vi "Get Tx IPs and Ports.vi"(0 "Target Names":string[](array[string])=["AE-HIL-1", "AE-HIL-2", "AE-HIL-3"], 1 "IP Addresses":string[](array[string])=["169.254.239.43", "169.254.184.119", "169.254.184.0"], 7 "Remote Target Name":string="AE-HIL-2", 13 "Local Target Index":i32) -> (4 "Local IP Address":string="169.254.239.43", 6 "Local Port Number":string="1000", 10 "Remote IP Address":string, 15 "Remote Port Number":string="1000")   [LabVIEW 2023]
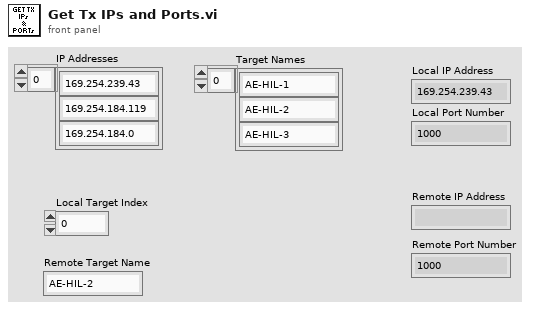
[diagram p1: front panel]
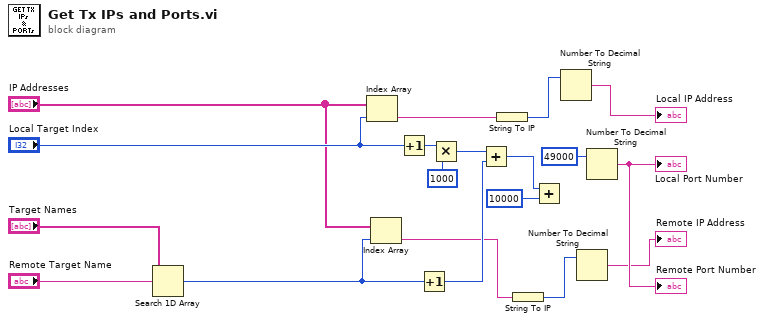
[diagram p0: block diagram]
diagram:
  n1 = Search 1D Array(1D array="Target Names", element="Remote Target Name") -> (index of element=w11:i32)  [unwired: 1 in]
  n2 = Index Array(array="IP Addresses", index="Local Target Index") -> (element=w7:string)
  n3 = Index Array(array="IP Addresses", index=w11) -> (element=w3:string)
  n4 = Increment(x="Local Target Index") -> (x+1=w12:i32)
  n5 = Increment(x=w11) -> (x+1=w14:i32)
  n6 = Multiply(x=w12, y=1000) -> (x*y=w15:i32)
  n7 = Add(x=w15, y=w14) -> (x+y=w9:i32)
  n8 = String To IP(1:w7) -> (0:w6:u32)
  n9 = String To IP(1:w3) -> (0:w4:u32)
  n10 = Add(x=w9, y=10000) -> ()  [unwired: 1 out]
  n11 = Number To Decimal String(number=w6) -> (decimal integer string=→"Local IP Address":string)  [unwired: 1 in]
  n12 = Number To Decimal String(number=w4) -> (decimal integer string=→"Remote IP Address":string)  [unwired: 1 in]
  n13 = Number To Decimal String(number=49000) -> (decimal integer string=→"Local Port Number" →"Remote Port Number":string)  [unwired: 1 in]
